vi "Write Name.vi"(8 "error in (no error)":errorcluster, 10 "Name":string, 11 "Sequence in":refnum<class "Sequence Config.lvclass">) -> (0 "error out":errorcluster, 3 "Sequence out":refnum<class "Sequence Config.lvclass">)   [LabVIEW 2015, in "Sequence Config.lvclass"]
uses:
  Sequence Config.lvclass
  Sequence Config.lvclass/Sequence Config.ctl
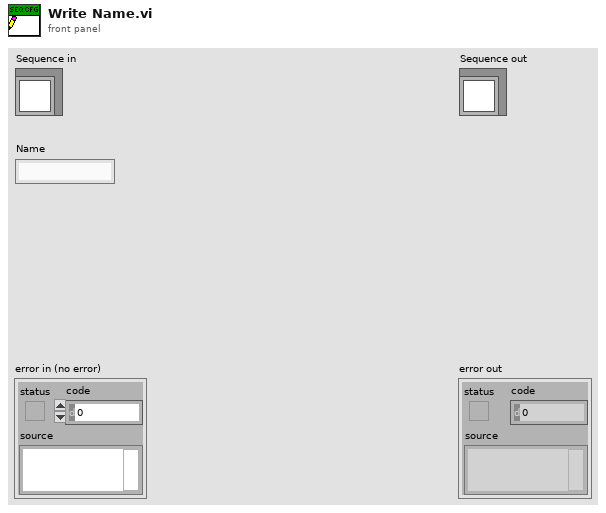
[diagram p1: front panel]
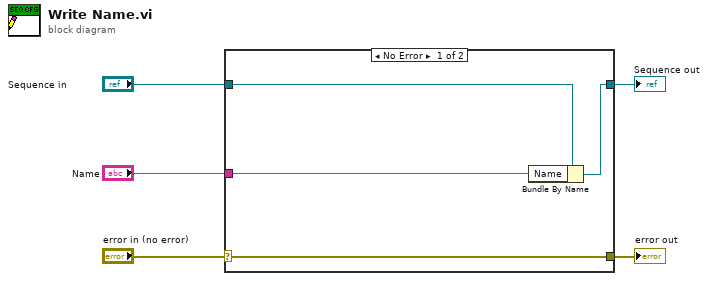
[diagram p0: block diagram]
diagram:
  n1 = case shown="No Error" "error in (no error)" {
    selector: "error in (no error)" -> [w9 w10]
    tunnel: [w9 w10] -> w4
    tunnel: [w7 w11] -> w2
    tunnel: "Sequence in" -> [w8 w11]
    tunnel: "Name" -> [w6 _]
    frame No Error {
      n2 = Bundle By Name(cluster=w8, "Name"=w6) -> (w7:refnum<class "Sequence Config.lvclass">)
    }
    frame Error {
    }
  }
  "error out" <- w4
  "Sequence out" <- w2
